vi "Write Table To XL sample.vi"(0 "Table":string[][](table)=[["", "", "", "", "", "", "", "", "", ""], ["", "", "", "", "", "", "", "", "", ""], ["", "", "", "", "", "", "", "", "", ""], ["", "", "", "", "", "", "", "", "", ""]], 2 "Filename":string="c:\\file", 4 "Completion Task":u16(ring) items=["Leave Excel Open", "Close Spreadsheet"]) -> ()   [LabVIEW 2010]
doc: "This VI demonstrates the basic idea of using the OLE Automation VIs by writing a Table into an Excel WorkSheet."
panel:
  in  "Excel._Worksheet":refnum<k7>
  in  "Excel._Application":refnum<k7>
  # "This VI demostrates the basic steps needed to enter the values in a table into a spreadsheet and then save it to a file."
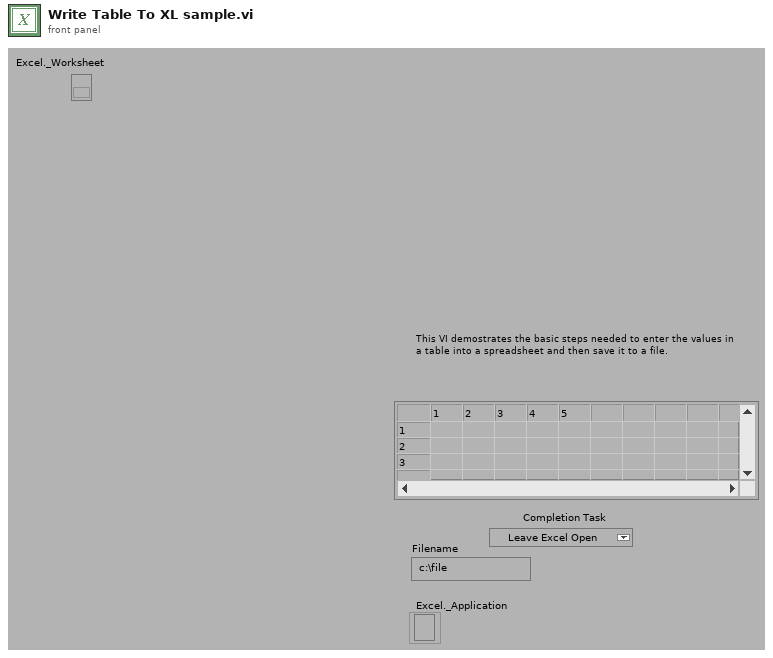
[diagram p1: front panel]
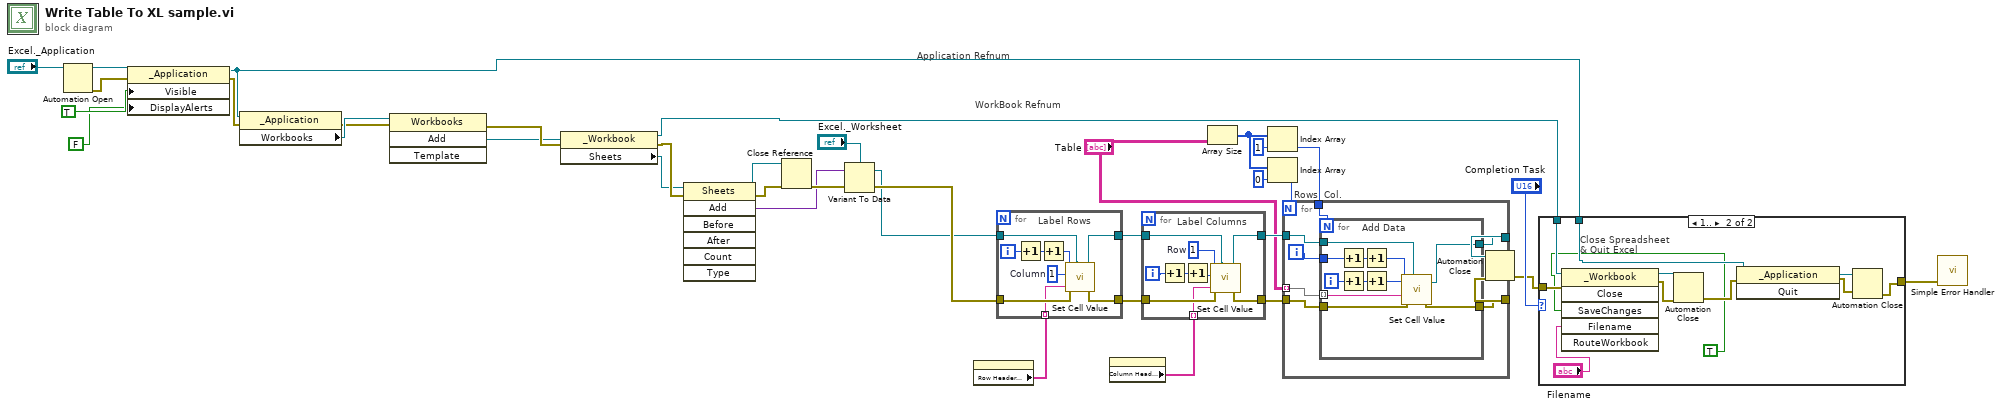
[diagram p0: block diagram]
diagram:
  # "Col."
  # "Rows"
  # "WorkBook Refnum"
  # "Application Refnum"
  n1 = Automation Open(Automation Refnum="Excel._Application") -> (Automation Refnum=w20:refnum<k7>, error out=w21:errorcluster)  [unwired: 3 in]
  n2 = property class="_Application"(reference=w20, error in=w21, "Visible"=TRUE, "DisplayAlerts"=FALSE) -> (reference out=w17:refnum<k7>, error out=w16:errorcluster)
  n3 = property class="_Application"(reference=w17, error in=w16) -> (error out=w14:errorcluster, "Workbooks"=w15:refnum<k7>)  [unwired: 1 out]
  n4 = invoke class="Workbooks" method="Add"(reference=w15, error in=w14) -> (error out=w13:errorcluster, "Add"=w12:refnum<k7>)  [unwired: 2 in, 2 out]
  n5 = property class="_Workbook"(reference=w12, error in=w13) -> (reference out=w4:refnum<k7>, error out=w11:errorcluster, "Sheets"=w3:refnum<k7>)
  n6 = invoke class="Sheets" method="Add"(reference=w3, error in=w11) -> (reference out=w9:refnum<k7>, error out=w10:errorcluster, "Add"=w5:variant)  [unwired: 5 in, 4 out]
  n7 = Close Reference(reference=w9, error in (no error)=w10) -> (error out=w8:errorcluster)
  n8 = Variant To Data(error in=w8, Variant=w5, type="Excel._Worksheet") -> (error out=w6:errorcluster, data=w2:refnum<k7>)
  n9 = property on="Property Node" class="Tbl (strict)"() -> ("Row Header Strings[]"=w35:string[])  [unwired: 2 in, 2 out]
  n10 = for {
    tunnel: w2 -> [w43]
    tunnel: w6 -> [w42]
    tunnel: [w41] -> w32
    tunnel: [w40] -> w33
    tunnel: w35 -> [w39] mode=indexing
    i -> [w47]
    w45 = 1  # Column
    # "Label Rows"
    n11 = Increment(x=w47) -> (x+1=w46:i32)
    n12 = Increment(x=w46) -> (x+1=w44:i32)
    n13 = call "Set Cell Value.vi"("Row"=w44, "Col"=w45, "Value"=w39, "error in (no error)"=w42, "Excel._Worksheet"=w43) -> ("Excel._Worksheet"=w40:refnum<k7>, "error out"=w41:errorcluster)
  }
  n14 = property on="Table" class="Tbl (strict)"() -> ("Column Header Strings[]"=w34:string[])  [unwired: 2 in, 2 out]
  n15 = for {
    tunnel: w33 -> [w54]
    tunnel: w32 -> [w53]
    tunnel: [w52] -> w30
    tunnel: [w51] -> w31
    tunnel: w34 -> [w48] mode=indexing
    i -> [w56]
    w49 = 1  # Row
    # "Label Columns"
    n16 = Increment(x=w56) -> (x+1=w55:i32)
    n17 = Increment(x=w55) -> (x+1=w50:i32)
    n18 = call "Set Cell Value.vi"("Row"=w49, "Col"=w50, "Value"=w48, "error in (no error)"=w53, "Excel._Worksheet"=w54) -> ("Excel._Worksheet"=w51:refnum<k7>, "error out"=w52:errorcluster)
  }
  n19 = Array Size(array="Table") -> (size(s)=w38:i32[])
  n20 = Index Array(array=w38, index=1) -> (element=w29:i32)
  n21 = Index Array(array=w38, index=0) -> (element=w28:i32)
  n22 = for {
    N: w28 -> [_]
    tunnel: w31 -> [w63]
    tunnel: w30 -> [w60]
    tunnel: [w62] -> w26
    tunnel: "Table" -> [w59] mode=indexing
    tunnel: w29 -> [w58]
    tunnel: [w57] -> w24
    i -> [w61]
    n23 = for {
      N: w58 -> [_]
      tunnel: w63 -> [w69]
      tunnel: w60 -> [w68]
      tunnel: [w67] -> w62
      tunnel: w61 -> [w66]
      tunnel: w59 -> [w65] mode=indexing
      tunnel: [w64] -> w57
      i -> [w74]
      # "Add Data"
      n24 = Increment(x=w66) -> (x+1=w73:i32)
      n25 = Increment(x=w74) -> (x+1=w71:i32)
      n26 = Increment(x=w73) -> (x+1=w72:i32)
      n27 = Increment(x=w71) -> (x+1=w70:i32)
      n28 = call "Set Cell Value.vi"("Row"=w72, "Col"=w70, "Value"=w65, "error in (no error)"=w68, "Excel._Worksheet"=w69) -> ("Excel._Worksheet"=w64:refnum<k7>, "error out"=w67:errorcluster)
    }
  }
  n29 = Automation Close(3:w26, 5:w24) -> (0:w25:errorcluster)
  n30 = case shown="1.." "Completion Task" {
    tunnel: [w75 w78] -> w22
    tunnel: w4 -> [_ w86]
    tunnel: w17 -> [_ w82]
    tunnel: w25 -> [w75 w85]
    frame ..0 {
    }
    frame 1.. {
      # "Close Spreadsheet\n& Quit Excel"
      n31 = invoke class="_Workbook" method="Close"(reference=w86, error in=w85, "SaveChanges"=TRUE, "Filename"="Filename") -> (reference out=w84:refnum<k7>, error out=w83:errorcluster)  [unwired: 2 in, 4 out]
      n32 = Automation Close(3:w83, 5:w84) -> (0:w81:errorcluster)
      n33 = invoke class="_Application" method="Quit"(reference=w82, error in=w81) -> (reference out=w79:refnum<k7>, error out=w80:errorcluster)  [unwired: 1 in, 1 out]
      n34 = Automation Close(3:w80, 5:w79) -> (0:w78:errorcluster)
    }
  }
  n35 = call <vilib>:"Simple Error Handler.vi"("error in (no error)"=w22) -> ()  [unwired: 4 in, 5 out]
